vi "Sub_Truncate_dataset.vi"(10 "Truncate data length":i32=5000, 11 "Experiment":T1={"Experimental Replay"={"Accelorometer"=array[210000 elements], "Displacement"=array[210000 elements], "dt"=0.0002, "Final Time"=42.0}, "Experimental Results"={"time_average_cycle"=0.0, "measured_frequency"=[], "date_time"="5/2/2024 1:10:00 PM", "estimated_pin_node"=[], "time_cycle_start"=[], "measured_pin_location"=[], "estimated_frequency"=[], "acceleration_data"=[], "accelerometer_sample_rate"=5000.0, "displacement_sample_rate"=5000.0, "time_compare_start"=array[564 elements], "time_subsample_start"=array[564 elements], "time_FEA_start"=array[564 elements], "time_FEA_end"=array[564 elements], "time_cycle_end"=array[564 elements], "time_accelerometer_aquire_start"=array[564 elements], "time_frequency_calculations_start"=array[564 elements], "time_frequency_calculations_end"=array[564 elements], "measured_pin_location_tt"=array[564 elements], "time_ACC_data_collection_start"=80808.5492656, "time_acceleration_data"=array[564 elements], "estimated_pin_location"=array[564 elements], "scaling_factor_Hz_per_pin_to_frequency_resolution"=nan, "Std_Dev_equale_particles_divided_3"=FALSE, "Auto_FFT_length"=FALSE, "windowed_acc_data"=array1x564[564 elements], "FFT"=array1x564[564 elements]}, "FEA Parameters"={"LEMP"={"Eigenvalues"=array[238 elements], "Square Transpose Eigenvectors"=array238x238[56644 elements], "1/deltaStiff"=1e-16}, "nodes of interest"=[19, 20, 21, 22, 23, 24, 25, 26, 27, 28, 29, 30, 31, 32, 33, 34, 35, 36, 37, 38, 39, 40, 41, 42, 43, 44, 45, 46, 47, 48, 49, 50, 51, 52], "all nodes"=[1, 2, 3, 4, 5, 6, 7, 8, 9, 10, 11, 12, 13, 14, 15, 16, 17, 18, 19, 20, 21, 22, 23, 24, 25, 26, 27, 28, 29, 30, 31, 32, 33, 34, 35, 36, 37, 38, 39, 40, 41, 42, 43, 44, 45, 46, 47, 48, 49, 50, 51, 52, 53, 54, 55, 56, 57, 58, 59, 60, 61, 62, 63, 64, 65, 66, 67, 68, 69, 70, 71, 72, 73, 74, 75, 76, 77, 78, 79, 80, 81, 82, 83, 84, 85, 86, 87, 88, 89, 90, 91, 92, 93, 94, 95, 96, 97, 98, 99, 100, 101, 102, 103, 104, 105, 106, 107, 108, 109, 110, 111, 112, 113, 114, 115, 116, 117, 118, 119], "Eigenvalue Method"=enum."0-Local Eigen Modification Procedure", "Mode Count"=3, "initial_pin_node"=0, "Sub Sample"=TRUE}, "Modeling Parameters"={"beam_length"=0.3525, "youngs_modulus"=209500000000.0, "torsion_spring"=0.0, "beam_height"=0.00635, "beam_width"=0.0508, "beam_density"=7900.0, "number_of_FEA_nodes"=120, "FFT_data_length"=4000, "standard_deviation"=2.0, "number_of_particles"=5, "min_FFT_power_value"=0.02, "initial_pin_node"=0, "accelerometer_mass"=0.055, "Max Roller Velocity"=3.32, "Max frequency delta per second"=-320.2269503546099, "Max frequency delta per node"=-1.0, "Min frequency"=49.84843481411623, "Max frequency"=87.165148551616}}) -> (3 "Experiment":T1)   [LabVIEW 2021]
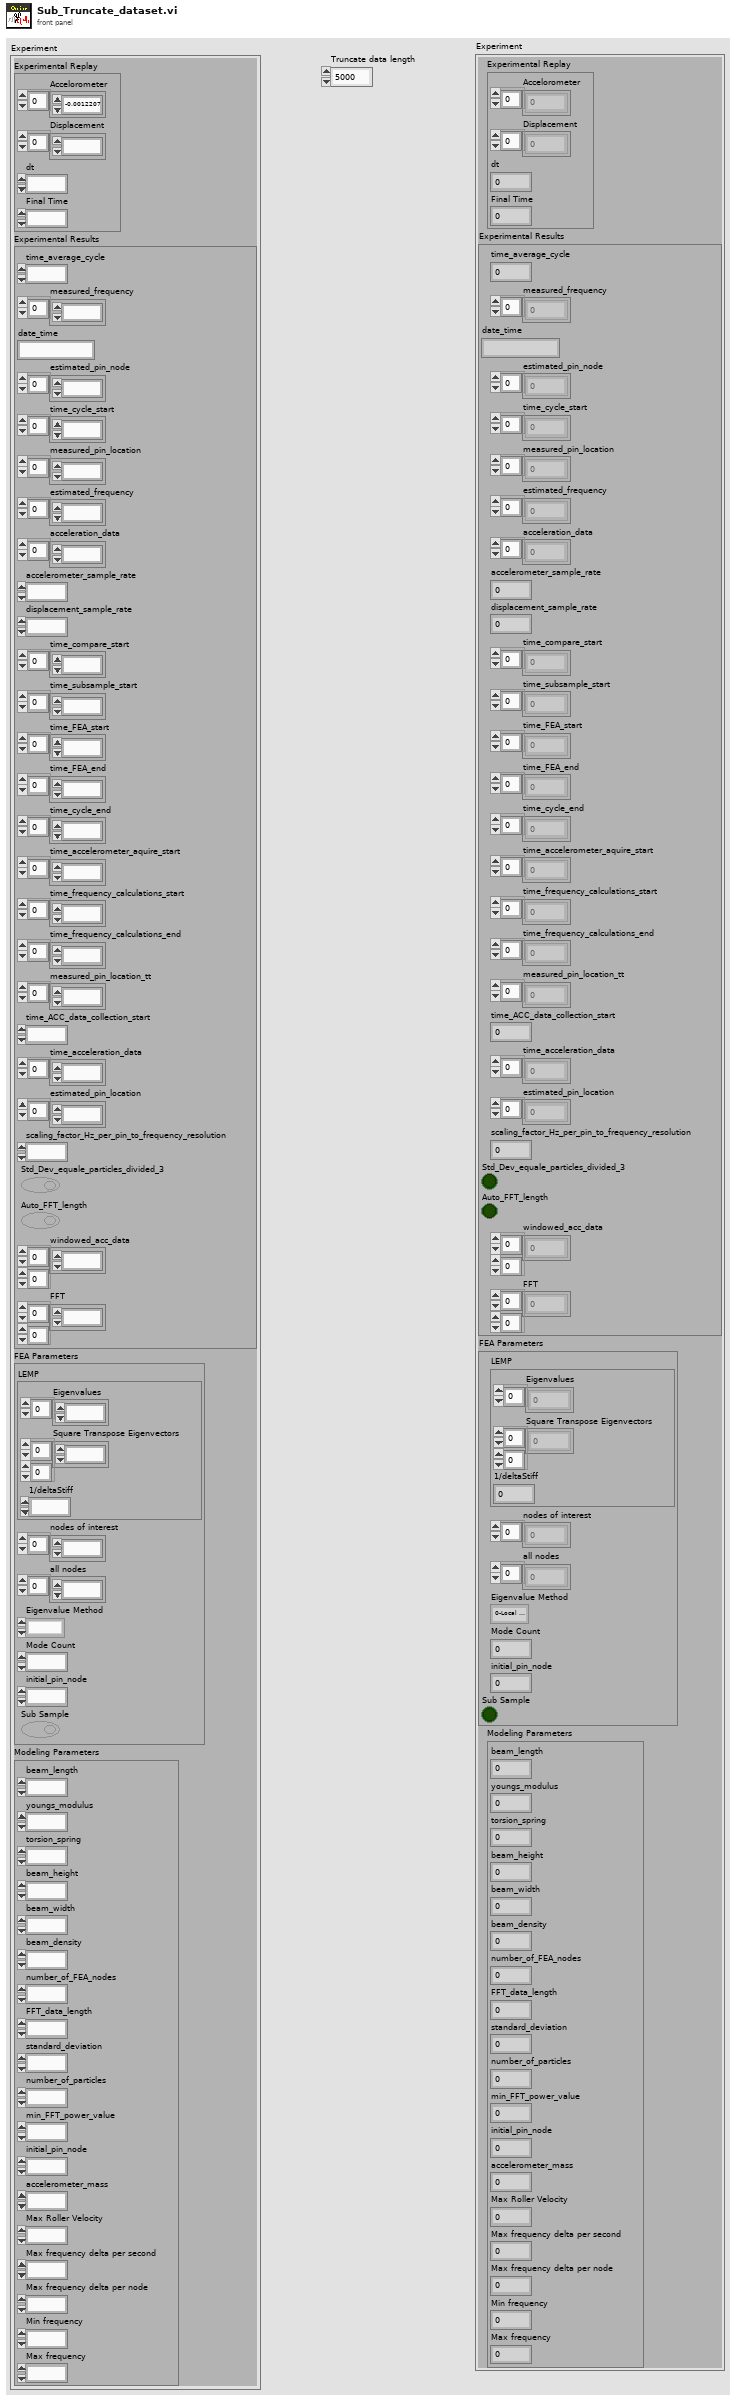
[diagram p1: front panel]
types:
  T1 = cluster{"Experimental Replay":cluster{"Accelorometer":dbl[], "Displacement":dbl[], "dt":dbl, "Final Time":dbl}, "Experimental Results":cluster{"time_average_cycle":dbl, "measured_frequency":dbl[], "date_time":string, "estimated_pin_node":i32[], "time_cycle_start":dbl[], "measured_pin_location":dbl[], "estimated_frequency":dbl[], "acceleration_data":dbl[], "accelerometer_sample_rate":dbl, "displacement_sample_rate":dbl, "time_compare_start":dbl[], "time_subsample_start":dbl[], "time_FEA_start":dbl[], "time_FEA_end":dbl[], "time_cycle_end":dbl[], "time_accelerometer_aquire_start":dbl[], "time_frequency_calculations_start":dbl[], "time_frequency_calculations_end":dbl[], "measured_pin_location_tt":dbl[], "time_ACC_data_collection_start":dbl, "time_acceleration_data":dbl[], "estimated_pin_location":dbl[], "scaling_factor_Hz_per_pin_to_frequency_resolution":dbl, "Std_Dev_equale_particles_divided_3":bool, "Auto_FFT_length":bool, "windowed_acc_data":dbl[][], "FFT":dbl[][]}, "FEA Parameters":cluster{"LEMP":cluster{"Eigenvalues":dbl[], "Square Transpose Eigenvectors":dbl[][], "1/deltaStiff":dbl}, "nodes of interest":i32[], "all nodes":i32[], "Eigenvalue Method":enum16{"0-Local Eigen Modification Procedure", "1-LabVIEW generalized eigenvalues", "2-LabVIEW M^-1K eigenvalues", "3-LabVIEW Cholesky Factorization", "4-Cholesky Factorization CPU SGL", "5-Cholesky Factorization CPU FXP", "6-Cholesky Factorization FPGA SGL", "7-Cholesky Factorization FPGA SGL SCL"}, "Mode Count":i32, "initial_pin_node":i32, "Sub Sample":bool}, "Modeling Parameters":cluster{"beam_length":dbl, "youngs_modulus":dbl, "torsion_spring":dbl, "beam_height":dbl, "beam_width":dbl, "beam_density":dbl, "number_of_FEA_nodes":i32, "FFT_data_length":i32, "standard_deviation":dbl, "number_of_particles":i32, "min_FFT_power_value":dbl, "initial_pin_node":i32, "accelerometer_mass":dbl, "Max Roller Velocity":dbl, "Max frequency delta per second":dbl, "Max frequency delta per node":dbl, "Min frequency":dbl, "Max frequency":dbl}}
  T2 = cluster{"Accelorometer":dbl[], "Displacement":dbl[], "dt":dbl, "Final Time":dbl}
  T3 = cluster{"time_average_cycle":dbl, "measured_frequency":dbl[], "date_time":string, "estimated_pin_node":i32[], "time_cycle_start":dbl[], "measured_pin_location":dbl[], "estimated_frequency":dbl[], "acceleration_data":dbl[], "accelerometer_sample_rate":dbl, "displacement_sample_rate":dbl, "time_compare_start":dbl[], "time_subsample_start":dbl[], "time_FEA_start":dbl[], "time_FEA_end":dbl[], "time_cycle_end":dbl[], "time_accelerometer_aquire_start":dbl[], "time_frequency_calculations_start":dbl[], "time_frequency_calculations_end":dbl[], "measured_pin_location_tt":dbl[], "time_ACC_data_collection_start":dbl, "time_acceleration_data":dbl[], "estimated_pin_location":dbl[], "scaling_factor_Hz_per_pin_to_frequency_resolution":dbl, "Std_Dev_equale_particles_divided_3":bool, "Auto_FFT_length":bool, "windowed_acc_data":dbl[][], "FFT":dbl[][]}
  T4 = cluster{"LEMP":cluster{"Eigenvalues":dbl[], "Square Transpose Eigenvectors":dbl[][], "1/deltaStiff":dbl}, "nodes of interest":i32[], "all nodes":i32[], "Eigenvalue Method":enum16{"0-Local Eigen Modification Procedure", "1-LabVIEW generalized eigenvalues", "2-LabVIEW M^-1K eigenvalues", "3-LabVIEW Cholesky Factorization", "4-Cholesky Factorization CPU SGL", "5-Cholesky Factorization CPU FXP", "6-Cholesky Factorization FPGA SGL", "7-Cholesky Factorization FPGA SGL SCL"}, "Mode Count":i32, "initial_pin_node":i32, "Sub Sample":bool}
  T5 = cluster{"beam_length":dbl, "youngs_modulus":dbl, "torsion_spring":dbl, "beam_height":dbl, "beam_width":dbl, "beam_density":dbl, "number_of_FEA_nodes":i32, "FFT_data_length":i32, "standard_deviation":dbl, "number_of_particles":i32, "min_FFT_power_value":dbl, "initial_pin_node":i32, "accelerometer_mass":dbl, "Max Roller Velocity":dbl, "Max frequency delta per second":dbl, "Max frequency delta per node":dbl, "Min frequency":dbl, "Max frequency":dbl}
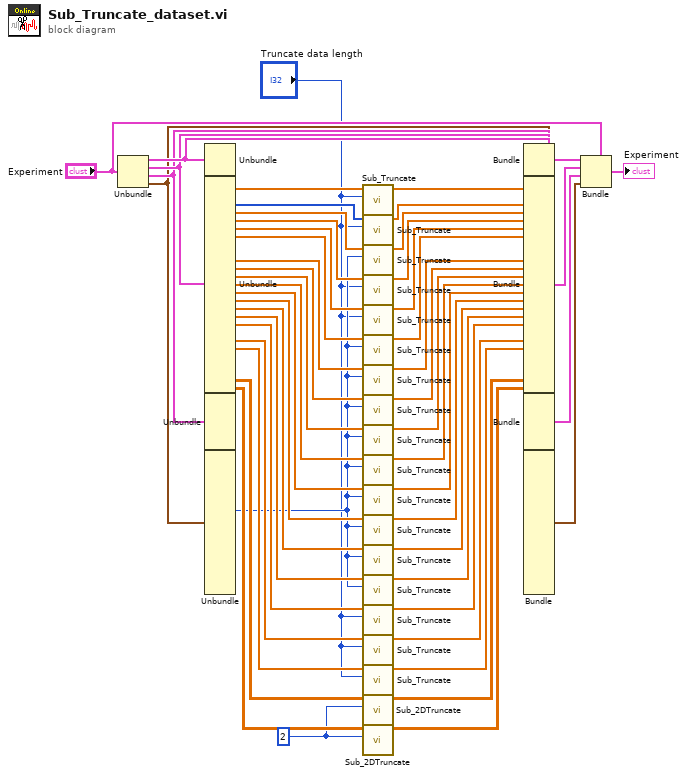
[diagram p0: block diagram]
diagram:
  w3 = 2
  n1 = Unbundle("Experiment") -> ("Experimental Replay"=w32:T2, "Experimental Results"=w31:T3, "FEA Parameters"=w30:T4, "Modeling Parameters"=w29:T5)
  n2 = Unbundle(w32) -> ()  [unwired: 4 out]
  n3 = Unbundle(w31) -> ("measured_frequency"=w51:dbl[], "estimated_pin_node"=w50:i32[], "time_cycle_start"=w49:dbl[], "measured_pin_location"=w48:dbl[], "estimated_frequency"=w47:dbl[], "acceleration_data"=w46:dbl[], "time_compare_start"=w45:dbl[], "time_subsample_start"=w44:dbl[], "time_FEA_start"=w43:dbl[], "time_FEA_end"=w42:dbl[], "time_cycle_end"=w41:dbl[], "time_accelerometer_aquire_start"=w40:dbl[], "time_frequency_calculations_start"=w39:dbl[], "time_frequency_calculations_end"=w38:dbl[], "measured_pin_location_tt"=w37:dbl[], "time_acceleration_data"=w36:dbl[], "estimated_pin_location"=w35:dbl[], "windowed_acc_data"=w34:dbl[][], "FFT"=w33:dbl[][])  [unwired: 8 out]
  n4 = Unbundle(w30) -> ()  [unwired: 7 out]
  n5 = Unbundle(w29) -> ("FFT_data_length"=w2:i32)  [unwired: 17 out]
  n6 = call "Sub_Truncate.vi"("samples"="Truncate data length", "array"=w51) -> ("array"=w28:dbl[])  [unwired: 9 in]
  n7 = call "Sub_Truncate.vi"("samples"="Truncate data length", "array"=w50) -> ("array"=w27:dbl[])  [unwired: 9 in]
  n8 = call "Sub_Truncate.vi"("samples"=w2, "array"=w49) -> ("array"=w26:dbl[])  [unwired: 9 in]
  n9 = call "Sub_Truncate.vi"("samples"="Truncate data length", "array"=w48) -> ("array"=w25:dbl[])  [unwired: 9 in]
  n10 = call "Sub_Truncate.vi"("samples"="Truncate data length", "array"=w47) -> ("array"=w24:dbl[])  [unwired: 9 in]
  n11 = call "Sub_Truncate.vi"("samples"=w2, "array"=w46) -> ("array"=w23:dbl[])  [unwired: 9 in]
  n12 = call "Sub_Truncate.vi"("samples"=w2, "array"=w45) -> ("array"=w22:dbl[])  [unwired: 9 in]
  n13 = call "Sub_Truncate.vi"("samples"=w2, "array"=w44) -> ("array"=w21:dbl[])  [unwired: 9 in]
  n14 = call "Sub_Truncate.vi"("samples"=w2, "array"=w43) -> ("array"=w20:dbl[])  [unwired: 9 in]
  n15 = call "Sub_Truncate.vi"("samples"=w2, "array"=w42) -> ("array"=w19:dbl[])  [unwired: 9 in]
  n16 = call "Sub_Truncate.vi"("samples"=w2, "array"=w41) -> ("array"=w18:dbl[])  [unwired: 9 in]
  n17 = call "Sub_Truncate.vi"("samples"=w2, "array"=w40) -> ("array"=w17:dbl[])  [unwired: 9 in]
  n18 = call "Sub_Truncate.vi"("samples"=w2, "array"=w39) -> ("array"=w16:dbl[])  [unwired: 9 in]
  n19 = call "Sub_Truncate.vi"("samples"=w2, "array"=w38) -> ("array"=w15:dbl[])  [unwired: 9 in]
  n20 = call "Sub_Truncate.vi"("samples"="Truncate data length", "array"=w37) -> ("array"=w14:dbl[])  [unwired: 9 in]
  n21 = call "Sub_Truncate.vi"("samples"="Truncate data length", "array"=w36) -> ("array"=w13:dbl[])  [unwired: 9 in]
  n22 = call "Sub_Truncate.vi"("samples"="Truncate data length", "array"=w35) -> ("array"=w12:dbl[])  [unwired: 9 in]
  n23 = call "Sub_2DTruncate.vi"("samples"=w3, 11:w34) -> ("array"=w11:dbl[][])  [unwired: 9 in]
  n24 = call "Sub_2DTruncate.vi"("samples"=w3, 11:w33) -> ("array"=w10:dbl[][])  [unwired: 9 in]
  n25 = Bundle(cluster=w32) -> (w9:T2)  [unwired: 4 in]
  n26 = Bundle(cluster=w31, "measured_frequency"=w28, "estimated_pin_node"=w27, "time_cycle_start"=w26, "measured_pin_location"=w25, "estimated_frequency"=w24, "acceleration_data"=w23, "time_compare_start"=w22, "time_subsample_start"=w21, "time_FEA_start"=w20, "time_FEA_end"=w19, "time_cycle_end"=w18, "time_accelerometer_aquire_start"=w17, "time_frequency_calculations_start"=w16, "time_frequency_calculations_end"=w15, "measured_pin_location_tt"=w14, "time_acceleration_data"=w13, "estimated_pin_location"=w12, "windowed_acc_data"=w11, "FFT"=w10) -> (w8:T3)  [unwired: 8 in]
  n27 = Bundle(cluster=w30) -> (w7:T4)  [unwired: 7 in]
  n28 = Bundle(cluster=w29) -> (w6:T5)  [unwired: 18 in]
  n29 = Bundle(cluster="Experiment", "Experimental Replay"=w9, "Experimental Results"=w8, "FEA Parameters"=w7, "Modeling Parameters"=w6) -> (→"Experiment":T1)
